vi "Get DI_group historian from PGserver.vi"(4 "time_min":timestamp, 6 "time_max":timestamp, 9 "conninfo":T1={"host"="localhost", "port"="5432", "client_encoding"="WIN1251", "dbname"="data", "user"="postgres", "password"=""}, 10 "ParamColumns":string[](array[string])=["EPBP1_XQ01", "EPBP2_XQ01", "EPBP3_XQ01"], 11 "ParamTable":string="EP_XQ.1802") -> (0 "error out":errorcluster, 3 "Array":cluster{timestamp[], bool[]}[](array[cluster]))   [LabVIEW 2019, in "Inputs.lvlib"]
uses:
  Database/ctl/Coninfo.ctl
  Database/PostgreSQL2LabVIEW/libpqlv/src/PQfinish.vi
  Database/PostgreSQL2LabVIEW/libpqlv/src/PQconnectdb.vi
  Database/PostgreSQL2LabVIEW/libpqlv/src/PQerrorMessage.vi
  Database/PostgreSQL2LabVIEW/libpqlv/src/PQstatus.vi
  <vilib>/dlg_ctls.llb/Space Constant.vi
  Database/PostgreSQL2LabVIEW/libpqlv/src/PQgetResult.vi
  Database/PostgreSQL2LabVIEW/libpqlv/src/PQclear.vi
  Database/PostgreSQL2LabVIEW/libpqUtility/src/PQfetchResultDataNotrans.vi
  Database/PostgreSQL2LabVIEW/libpqlv/src/PQresultErrorMessage.vi
  Database/PostgreSQL2LabVIEW/libpqlv/src/PQresultStatus.vi
  Database/PostgreSQL2LabVIEW/libpqlv/src/PQsendQuery.vi
  Database/PostgreSQL2LabVIEW/libpqlv/src/PQnfields.vi
  Database/PostgreSQL2LabVIEW/libpqlv/src/PQntuples.vi
  Database/PostgreSQL2LabVIEW/libpqlv/src/PQgetvalue.vi
  Inputs.lvlib
  Database/PostgreSQL2LabVIEW/libpqUtility/libpqutility.lvlib
  Database/PostgreSQL.lvlib
panel:
  out "PQStatus":T2(ring)
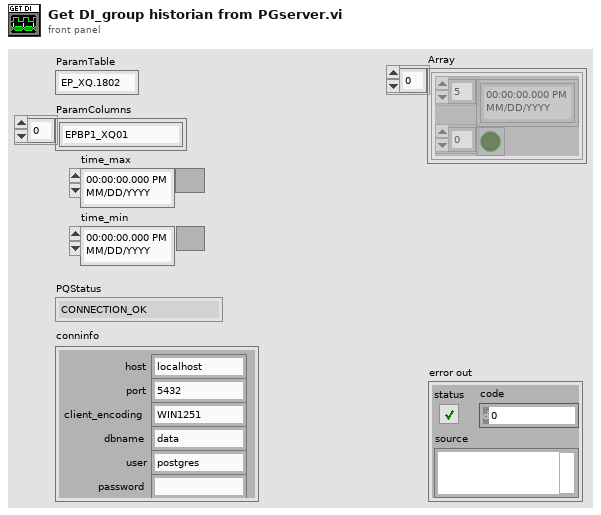
[diagram p1: front panel]
types:
  T1 = typedef "PostgreSQL.lvlib/Coninfo.ctl" = cluster{"host":string, "port":string, "client_encoding":string, "dbname":string, "user":string, "password":string}
  T2 = enum32{"CONNECTION_OK", "CONNECTION_BAD", "CONNECTION_STARTED", "CONNECTION_MADE", "CONNECTION_AWAITING_RESPONSE", "CONNECTION_AUTH_OK", "CONNECTION_SETENV", "CONNECTION_SSL_STARTUP", "CONNECTION_NEEDED"}
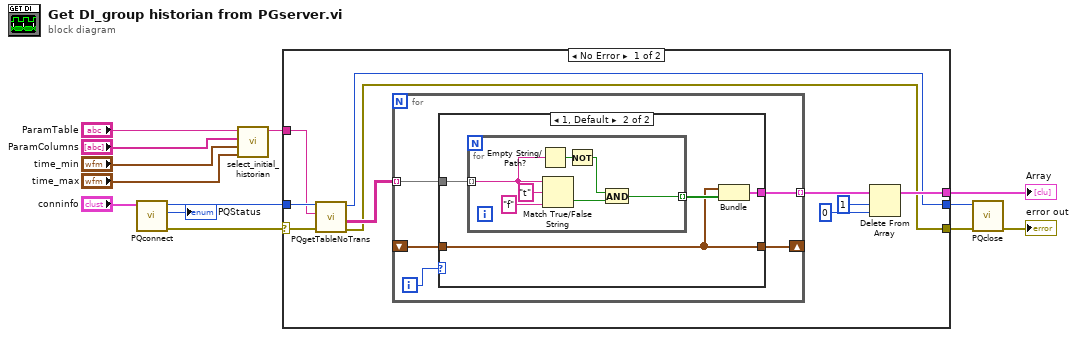
[diagram p0: block diagram]
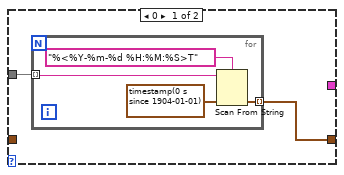
[diagram p2: hidden frame]
diagram:
  n1 = call "PQconnect.vi"("conninfo"="conninfo") -> ("error out"=w13:errorcluster, "PQStatus"=→"PQStatus":T2, "conn"=w2:u32)  [unwired: 8 in]
  n2 = call "select_initial_historian.vi"("time_max"="time_max", "time_min"="time_min", "Column table"="ParamColumns", "table"="ParamTable") -> ("parameters"=w3:string)  [unwired: 7 in]
  n3 = case shown="No Error" w13 {
    selector: w13 -> [w18 w47]
    tunnel: [w20 _] -> w12
    tunnel: w2 -> [w19 w46]
    tunnel: w3 -> [w17 _]
    tunnel: [w15 w47] -> w9
    tunnel: [w14 w46] -> w1
    frame No Error {
      n4 = call "PQgetTableNoTrans.vi"("error in"=w18, "query"=w17, "conn"=w19) -> ("error out"=w15:errorcluster, "Data"=w16:string[][], "conn_out"=w14:u32)  [unwired: 4 in, 2 out]
      n5 = for {
        tunnel: [w27] -> w23 mode=indexing
        tunnel: w16 -> [w28] mode=indexing
        shift-right: [w26] -> _
        shift-left: _ -> [w25]
        i -> [w24]
        n6 = case shown="1, Default" w24 {
          tunnel: [w30 w35] -> w26
          tunnel: w28 -> [w29 w38]
          tunnel: [_ w36] -> w27
          tunnel: w25 -> [_ w35]
          frame 0 {
            n7 = for {
              tunnel: [w31] -> w30 mode=indexing
              tunnel: w29 -> [w32] mode=indexing
              n8 = Scan From String(format string="%<%Y-%m-%d %H:%M:%S>T" ("string"), input string=w32, default 1=timestamp(0 s since 1904-01-01) ("time stamp")) -> (output 1=w31:timestamp)  [unwired: 2 in, 3 out]
            }
          }
          frame 1, Default {
            n9 = for {
              tunnel: w38 -> [w43] mode=indexing
              tunnel: [w39] -> w37 mode=indexing
              n10 = Empty String/Path?(string/path=w43) -> (empty?=w42:bool)
              n11 = Match True/False String(2:"f" ("false string"), 3:"t" ("true string"), 4:w43) -> (0:w40:bool)  [unwired: 1 out]
              n12 = Not(x=w42) -> (.not. x?=w41:bool)
              n13 = And(x=w41, y=w40) -> (x .and. y?=w39:bool)
            }
            n14 = Bundle(w35, w37) -> (w36:cluster{timestamp[], bool[]})  [unwired: 1 in]
          }
        }
      }
      n15 = Delete From Array(array=w23, length=1, index=0) -> (array with subset deleted=w20:cluster{timestamp[], bool[]}[])  [unwired: 1 out]
    }
    frame Error {
    }
  }
  "Array" <- w12
  n16 = call "PQclose.vi"("error in (no error)"=w9, "conn"=w1) -> ("error out"=→"error out":errorcluster)  [unwired: 9 in]
